vi "init_hw.vi"(8 "error in (no error)":errorcluster, 11 "dummyStage in":refnum<class "dummyStage.lvclass">) -> (0 "error out":errorcluster, 2 "Boolean":bool=TRUE, 3 "dummyStage out":refnum<class "dummyStage.lvclass">)   [LabVIEW 2019, in "dummyStage.lvlib" / "dummyStage.lvclass"]
uses:
  dummyStage.lvclass
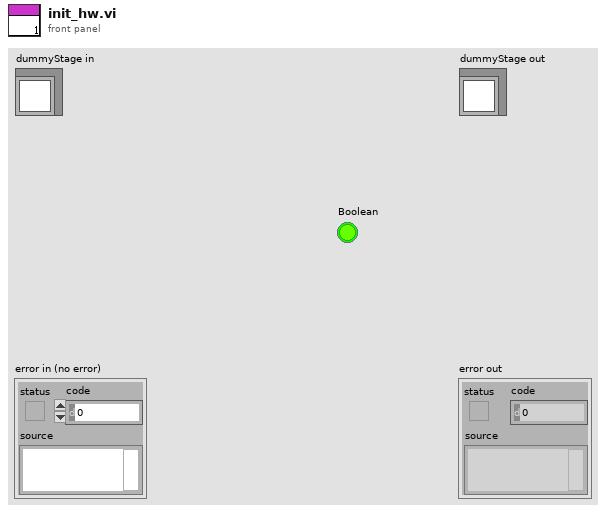
[diagram p1: front panel]
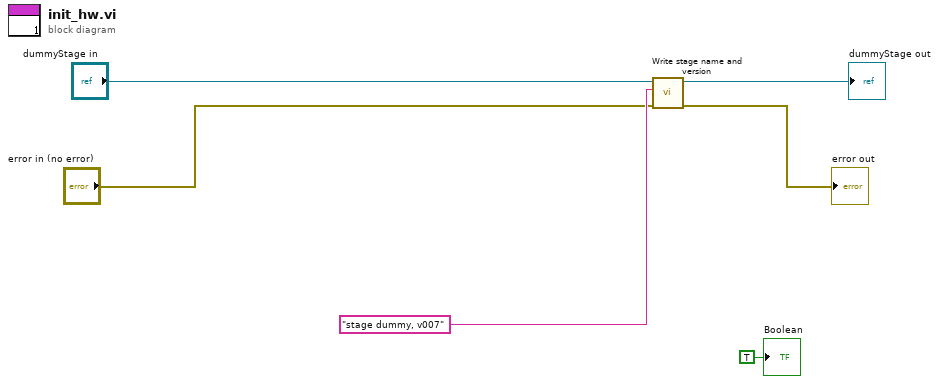
[diagram p0: block diagram]
diagram:
  n1 = call-dynamic "Write stage name and version.vi"("error in (no error)"="error in (no error)", "stage name and version"="stage dummy, v007" ("stage name, version"), "_stage in"="dummyStage in") -> ("error out"=→"error out":errorcluster, "_stage out"=→"dummyStage out":refnum<class "dummyStage.lvclass">)  [unwired: 7 in]
  "Boolean" <- TRUE ("Boolean")
